vi "tm_setparameter.vi"(6 "View":i32, 8 "error in (no error)":errorcluster, 9 "Value in":dbl, 10 "Parameter":i32(ring)=1 items=["BINNING"=1, "BITS PER CHANNEL"=2, "ACTIVE VIEW INDEX"=3, "CCD MODE"=4, "SENSOR MODE"=5, "READOUT MODE"=6, "EXPOSURE TIME"=7, "CONTRAST GAIN"=8, "CONTRAST OFFSET"=9, "LIGHT MODE"=10, "SENSITIVITY"=11, "WHITE BALANCE"=12, "PHOTON IMAGING MODE"=13, "HIGH DYNAMIC RANGE MODE"=14, "TRIGGER SOURCE"=15, "TRIGGER ACTIVE"=16, "TRIGGER MODE"=17, "TRIGGER POLARITY"=18, "TRIGGER GLOBAL EXPOSURE"=19, "FIRST TRIGGER BEHAVIOR"=20, "TRIGGER TIMES"=21, "OUTPUT TRIGGER POLARITY"=22, "OUTPUT TRIGGER DELAY"=23, "OUTPUT TRIGGER PERIOD"=24, "TEMPERATURE"=25, "TEMPERATURE TARGET"=26, "SENSOR COOLER FAN"=27, "MECHANICAL SHUTTER"=28, "BACK FOCUS POSITION"=29, "FRAMEBUNDLE MODE"=30, "FRAMEBUNDLE NUMBER"=31, "LINEBUNDLE HEIGHT"=32, "TRIGGER CONNECTOR"=33, "IMAGE PIXEL TYPE"=34], 11 "Handle in":u32) -> (0 "error out":errorcluster, 3 "Handle out":u32)   [LabVIEW 2015]
uses:
  tmcamcon.dll
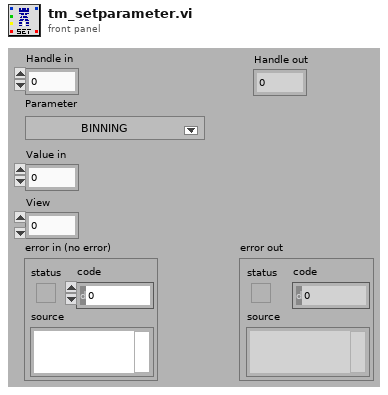
[diagram p1: front panel]
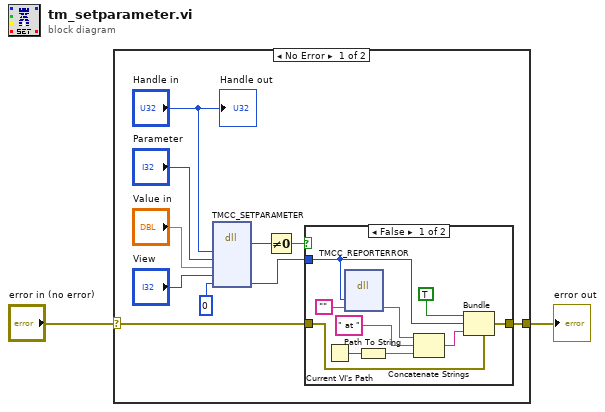
[diagram p0: block diagram]
diagram:
  n1 = case shown="No Error" "error in (no error)" {
    selector: "error in (no error)" -> [w8 w24]
    tunnel: [w5 w24] -> w1
    frame No Error {
      n2 = dll-call lib="tmcamcon.dll" fn="TMCC_SETPARAMETER"("HDCAM"="Handle in", "parameter"="Parameter", "value"="Value in", "view"="View", "Erval"=0) -> ("return type"=w12:u32, "Erval"=w7:i32)  [unwired: 7 in, 2 out]
      n3 = Not Equal To 0?(x=w12) -> (x != 0?=w6:bool)
      n4 = case shown="False" w6 {
        tunnel: w8 -> [w22 w23]
        tunnel: [w21 w23] -> w5
        tunnel: w7 -> [w15 _]
        frame False {
          n5 = Current VI's Path() -> (path=w20:path)
          n6 = dll-call lib="tmcamcon.dll" fn="TMCC_REPORTERROR"("error"=w15, "buf"="") -> ("buf"=w14:string)  [unwired: 5 in, 2 out]
          n7 = Path To String(path=w20) -> (string=w16:string)
          n8 = Concatenate Strings(w14, " at ", w16) -> (w19:string)
          n9 = Bundle(cluster=w22, "status"=TRUE, "code"=w15, "source"=w19) -> (w21:errorcluster)
        }
        frame True {
        }
      }
      "Handle out" <- "Handle in"
    }
    frame Error {
    }
  }
  "error out" <- w1
